vi "Is Tunnel Indexing.vi"(10 "Object Placement":enum32{"Choice 1", "Choice 2"}(radio), 11 "Tunnel Ref":refnum<vi>) -> (0 "Array Iinside":bool, 1 "Array outside":bool, 2 "Chosen Terminal is indexing":bool, 3 "Tunnel is indexing":bool, 4 "Non-Array Term":refnum<vi>, 5 "Array Term":refnum<vi>)   [LabVIEW 2023]
uses:
  <vilib>/Utility/Data Type/NI_Data Type.lvlib
  <userlib>/_OpenG.lib/error/error.llb/openg_error.lvlib
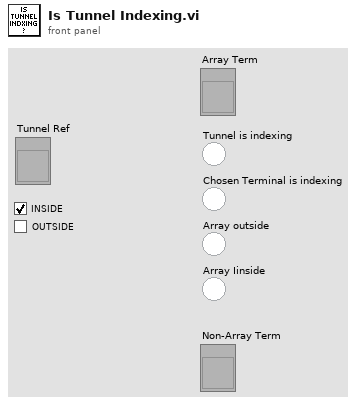
[diagram p1: front panel]
types:
  T1 = enum8{"Invalid Type", "Void", "I8", "I16", "I32", "I64", "U8", "U16", "U32", "U64", "Single Float", "Double Float", "Extended Float", "Single Complex", "Double Complex", "Extended Complex", "Enum U8", "Enum U16", "Enum U32", "Enum U64", "Single Float With Unit", "Double Float With Unit", "Extended Float With Unit", "Single Complex with Unit", "Double Complex with Unit", "Extended Complex with Unit", "Boolean", "String", "Path", "Picture", "Tag", "Array", "Cluster", "Variant", "LV Variant", "Waveform", "Timestamp", "Digital Waveform", "Digital Data", "ExpressData", "Refnum", "External Data", "VI", "Poly VI", "LabVIEW Class Instance", "Fixed Point"}
  T2 = typedef "NI_Data Type.lvlib/Data Type.ctl" = enum8{"Invalid Type", "Void", "I8", "I16", "I32", "I64", "U8", "U16", "U32", "U64", "Single Float", "Double Float", "Extended Float", "Single Complex", "Double Complex", "Extended Complex", "Enum U8", "Enum U16", "Enum U32", "Enum U64", "Single Float With Unit", "Double Float With Unit", "Extended Float With Unit", "Single Complex with Unit", "Double Complex with Unit", "Extended Complex with Unit", "Boolean", "String", "Path", "Picture", "Tag", "Array", "Cluster", "Variant", "LV Variant", "Waveform", "Timestamp", "Digital Waveform", "Digital Data", "ExpressData", "Refnum", "External Data", "VI", "Poly VI", "LabVIEW Class Instance", "Fixed Point", "Set Collection", "Map Collection"}
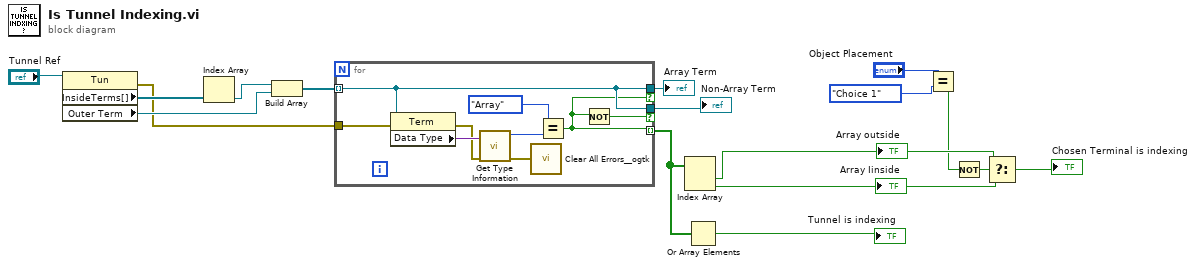
[diagram p0: block diagram]
diagram:
  n1 = property class="Tun"(reference="Tunnel Ref") -> (error out=w3:errorcluster, "InsideTerms[]"=w16:refnum<vi>[], "Outer Term"=w14:refnum<vi>)  [unwired: 1 in, 1 out]
  n2 = Index Array(array=w16) -> (element=w15:refnum<vi>)  [unwired: 1 in]
  n3 = Build Array(w15, w14) -> (w13:refnum<vi>[])
  n4 = for {
    tunnel: w13 -> [w20] mode=indexing
    tunnel: [w19] -> w5 mode=indexing
    tunnel: w3 -> [w21]
    tunnel: [w20] -> w2 if=w19
    tunnel: [w20] -> w1 if=w18
    n5 = property class="Term"(reference=w20, error in=w21) -> (error out=w23:errorcluster, "Data Type"=w26:variant)  [unwired: 1 out]
    n6 = call <vilib>:"Get Type Information.vi"("error in (no error)"=w23, "variant"=w26) -> ("error out"=w22:errorcluster, "type"=w25:T2)  [unwired: 5 in, 3 out]
    n7 = call <userlib>:"Clear All Errors__ogtk.vi"("Error In"=w22) -> ()  [unwired: 3 in, 1 out]
    n8 = Equal?(x=T1."Array" ("type"), y=w25) -> (x = y?=w19:bool)
    n9 = Not(x=w19) -> (.not. x?=w18:bool)
  }
  "Array Term" <- w2
  "Non-Array Term" <- w1
  n10 = Index Array(array=w5) -> (element #1=w10:bool, element #2=w9:bool)  [unwired: 2 in]
  "Array outside" <- w10
  "Array Iinside" <- w9
  n11 = Or Array Elements(Boolean array=w5) -> (logical OR=→"Tunnel is indexing":bool)
  n12 = Equal?(x="Object Placement", y=enum32{"Choice 1", "Choice 2"}."Choice 1" ("Object Placement")) -> (x = y?=w8:bool)
  n13 = Not(x=w8) -> (.not. x?=w6:bool)
  n14 = Select(t=w10, s=w6, f=w9) -> (s? t:f=→"Chosen Terminal is indexing":bool)
